vi "GetModuleDescriptions.vi"(7 "Operation":T1, 8 "Error In":errorcluster, 11 "Module Name In":string) -> (0 "Error Out":errorcluster, 2 "Found?":bool, 3 "Data Out":string)   [LabVIEW 2011]
doc: "This VI will store module descriptions."
uses:
  Controls/GetModueDescriptionsOperations.ctl
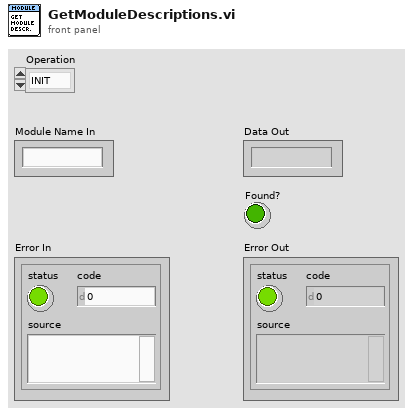
[diagram p1: front panel]
types:
  T1 = typedef "GetModueDescriptionsOperations.ctl" = enum16{"INIT", "GET"}
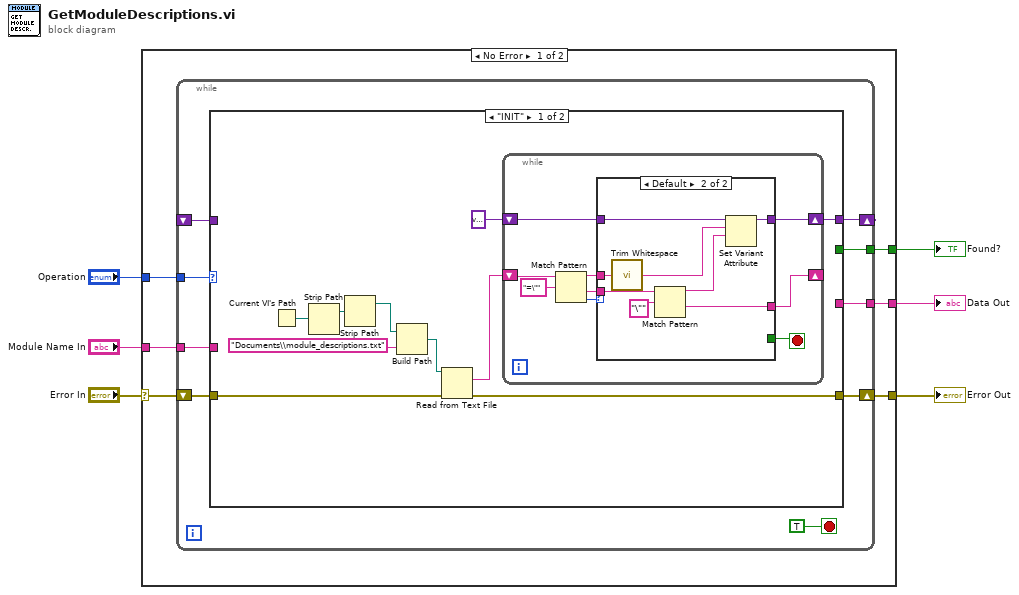
[diagram p0: block diagram]
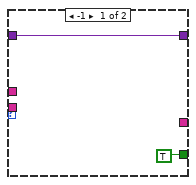
[diagram p2: hidden frame]
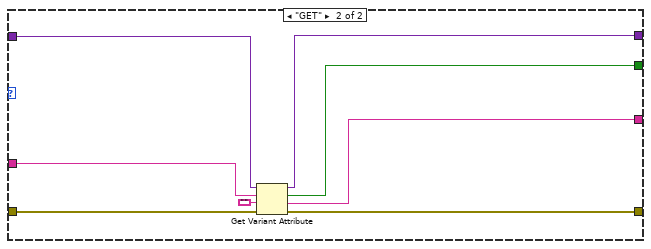
[diagram p3: hidden frame]
diagram:
  n1 = case shown="No Error" "Error In" {
    selector: "Error In" -> [w10 w59]
    tunnel: [w12 w59] -> w6
    tunnel: "Operation" -> [w11 _]
    tunnel: "Module Name In" -> [w9 _]
    tunnel: [w8 _] -> w2
    tunnel: [w7 _] -> w1
    frame No Error {
      n2 = while {
        shift-right: [w20] -> w12
        shift-left: w10 -> [w21]
        tunnel: w11 -> [w19]
        shift-right: [w18] -> _
        shift-left: _ -> [w17]
        tunnel: w9 -> [w16]
        tunnel: [w15] -> w8
        tunnel: [w14] -> w7
        stop <- TRUE stop-if-true
        n3 = case shown="\"INIT\"" w19 {
          tunnel: w21 -> [w24 w58]
          tunnel: [w23 w57] -> w20
          tunnel: [w22 w51] -> w18
          tunnel: w17 -> [_ w52]
          tunnel: w16 -> [_ w56]
          tunnel: [_ w54] -> w15
          tunnel: [_ w53] -> w14
          frame "INIT" {
            n4 = Current VI's Path() -> (path=w29:path)
            n5 = Strip Path(path=w29) -> (stripped path=w28:path)  [unwired: 1 out]
            n6 = Strip Path(path=w28) -> (stripped path=w27:path)  [unwired: 1 out]
            n7 = Build Path(base path=w27, name or relative path="Documents\\module_descriptions.txt") -> (appended path=w25:path)
            n8 = Read from Text File(file (use dialog)=w25, error in=w24) -> (text=w31:string, error out=w23:errorcluster)  [unwired: 2 in, 2 out]
            n9 = while {
              shift-right: [w32] -> _
              shift-left: w31 -> [w40]
              shift-right: [w37] -> w22
              shift-left: variant -> [w36]
              stop <- w33 stop-if-true
              n10 = Match Pattern(string=w40, regular expression="=\"") -> (before substring=w38:string, after substring=w35:string, offset past match=w34:i32)  [unwired: 1 in, 1 out]
              n11 = case shown="Default" w34 {
                tunnel: w38 -> [_ w50]
                tunnel: [w42 w49] -> w37
                tunnel: w36 -> [w42 w48]
                tunnel: w35 -> [_ w46]
                tunnel: [TRUE _] -> w33
                tunnel: [_ w44] -> w32
                frame -1 {
                }
                frame Default {
                  n12 = call <vilib>:"Trim Whitespace.vi"("string"=w50) -> ("trimmed string"=w47:string)  [unwired: 1 in]
                  n13 = Match Pattern(string=w46, regular expression="\"") -> (before substring=w43:string, after substring=w44:string)  [unwired: 1 in, 2 out]
                  n14 = Set Variant Attribute(Variant=w48, name=w47, value=w43) -> (Variant out=w49:variant)  [unwired: 1 in, 2 out]
                }
              }
            }
          }
          frame "GET" {
            n15 = Get Variant Attribute(Variant=w52, name=w56, default value (empty Variant)="" ("name"), error in=w58) -> (duplicate Variant=w51:variant, found=w54:bool, value=w53:string, error out=w57:errorcluster)
          }
        }
      }
    }
    frame Error {
    }
  }
  "Error Out" <- w6
  "Found?" <- w2
  "Data Out" <- w1
